vi "Pack6_UNDT.vi"(0 "data_in":u8[](array[numeric])=[86, 52, 18, 120, 86, 52, 18, 2, 0, 0, 0, 112, 204, 67, 22, 156, 119, 190, 97, 0, 16, 0, 139, 0, 0, 0, 0, 0, 0, 0, 0, 0, 0, 0, 0, 0, 0, 0, 0, 0, 0, 0, 0, 111, 18, 131, 57, 0, 0, 0, 0, 0, 1, 0, 1, 43, 25, 0, 1, 255, 255, 34, 34, 255, 255, 255, 255, 255, 255, 255, 255, 255, 255, 255, 255, 255, 255, 255, 255, 255, 255, 255, 255, 255, 255, 255, 255, 255, 255, 255, 255, 255, 255, 255, 255, 255, 255, 255, 255, 255, 255, 255, 255, 255, 255, 255, 255, 255, 255, 255, 255, 255, 255, 255, 255, 255, 255, 255, 255, 255, 255, 255, 255, 120, 86, 52, 18, 1, 0, 0, 0, 112, 204, 67, 22, 156, 119, 190, 97, 0, 16, 0, 139, 0, 0, 0, 0, 0, 0, 0, 0, 0, 0, 0, 0, 0, 0, 0, 0, 0, 0, 0, 0, 111, 18, 131, 57, 0, 0, 0, 0, 0, 1, 0, 1, 43, 25, 0, 1, 255, 255, 34, 17, 255, 255, 255, 255, 255, 255, 255, 255, 255, 255, 255, 255, 255, 255, 255, 255, 255, 255, 255, 255, 255, 255, 255, 255, 255, 255, 255, 255, 255, 255, 255, 255, 255, 255, 255, 255, 255, 255, 255, 255, 255, 255, 255, 255, 255, 255, 255, 255, 255, 255, 255, 255, 255, 255, 255, 255, 255, 255, 255] format="%02x", 1 "K_scale":dbl, 5 "N tick":u8 format="%02x", 9 "OptionPACK5":T4={"MagicWordStr"="xV4\u0012", "Header size"=56, "Проверка CRC8"=TRUE, "Проверка конца пакета"=TRUE, "GainCompens"=FALSE, "GainCorrection"=[[0.0, 1.0, 2.0, 3.0, 4.0, 5.0, 6.0, 7.0, 8.0, 9.0, 10.0, 11.0, 12.0, 13.0, 14.0, 15.0, 16.0, 17.0, 18.0, 19.0, 20.0, 21.0, 22.0, 23.0, 24.0, 25.0, 26.0, 27.0, 28.0, 29.0, 30.0, 31.0, 32.0, 33.0, 34.0, 35.0, 36.0, 37.0, 38.0, 39.0, 40.0], [0.007480379377256454, 0.05961025727668039, -0.2256445449069899, -0.08477459513390878, -0.19260677802883944, -0.022395839150075085, -0.076115384746043, -0.07452129161654766, -0.012380415371210218, 0.012737541388962995, 0.06895372697540661, 0.015013157866332921, -0.007045606467342559, -0.029720988817163698, 0.012859755243868034, 0.014783052645341199, 0.008698262907434648, -0.0007780407280235585, 0.0004171488690068028, 0.02092967406906331, 0.0018566195042745877, 0.009729465944000381, 0.007879136597780506, 0.028348095755020803, 0.01788279432686344, 0.01316889208220224, 0.008960543359635798, 0.01306464703510712, 0.03262709696783729, 0.0012714692473612531, -0.03761892820570949, -0.0316523389742032, 0.008159355326511571, 0.0081809109877908, 0.03836815904439456, 0.06681584703351648, 0.06544874790085742, 0.08623523673581365, 0.06010176834536063, 0.06195241245042141, 0.05245036073698361], [0.0, 0.0, 0.0, 0.0, 0.0, 0.0, 0.0, 0.0, 0.0, 0.0, 0.0, 0.0, 0.0, 0.0, 0.0, 0.0, 0.0, 0.0, 0.0, 0.0, 0.0, 0.0, 0.0, 0.0, 0.0, 0.0, 0.0, 0.0, 0.0, 0.0, 0.0, 0.0, 0.0, 0.0, 0.0, 0.0, 0.0, 0.0, 0.0, 0.0, 0.0]], "CorCh"=[], "Неотбрасывать BadEnd пакеты"=TRUE, "Неотбрасывать BadCRC пакеты"=TRUE} {"GainCorrection" format="%_4g"}, 11 "error in":errorcluster, 12 "Привести к 1":bool, 14 "GainCoef":bool) -> (3 "offset past match":i32=4, 4 "data_out":u8[](array[numeric]), 6 "output cluster 2":T2 {"UNDT_Cluster"."Gain Coeff" format="%#_6e"; "UNDT_Cluster"."Reserve 1" format="%02x"; "UNDT_Cluster"."Mux TX/RX" format="%02x"; "UNDT_Cluster"."ScanDelay" format="%02x"; "UNDT_Cluster"."SamplingInterval" format="%#_6e"; "UNDT_Cluster"."Lose Packet" format="%08x"; "UNDT_Cluster"."EncodersParam2" format="%016x"; "UNDT_Cluster"."EncodersParam1" format="%016x"; "UNDT_Cluster"."CRC 8" format="%02x"; "UNDT_Cluster"."N chanel" format="%02x"; "UNDT_Cluster"."N tick" format="%02x"; "UNDT_Cluster"."Ncycle" format="%04x"; "UNDT_Cluster"."FrameFormatVersion" format="%02x"; "UNDT_Cluster"."MagicWord" format="%.0x"}, 8 "Status":T1={"CRC8Good"=TRUE, "PackEndGood"=TRUE, "MWFind"=TRUE, "PackToSmall"=FALSE, "offset"=4}, 10 "PackToSmall":bool, 15 "error out":errorcluster)   [LabVIEW 2017]
uses:
  Control_EU/UNDT_ClusterPackRevers (Type).ctl
  Control_EU/DataCluster.ctl
  Control_EU/OptionPACK5.ctl
  Control_EU/Status_pack5.ctl
panel:
  out "magic_word":u8[](array[numeric])
  out "OfsetEndPack":i32
  out "MWFind":bool=TRUE
  out "Проверка конца пакета":bool=TRUE
  out "PackEndGood":bool=TRUE
  out "Проверка CRC8":bool=TRUE
  out "CRC8Good":bool=TRUE
  out "Header size":u32=56
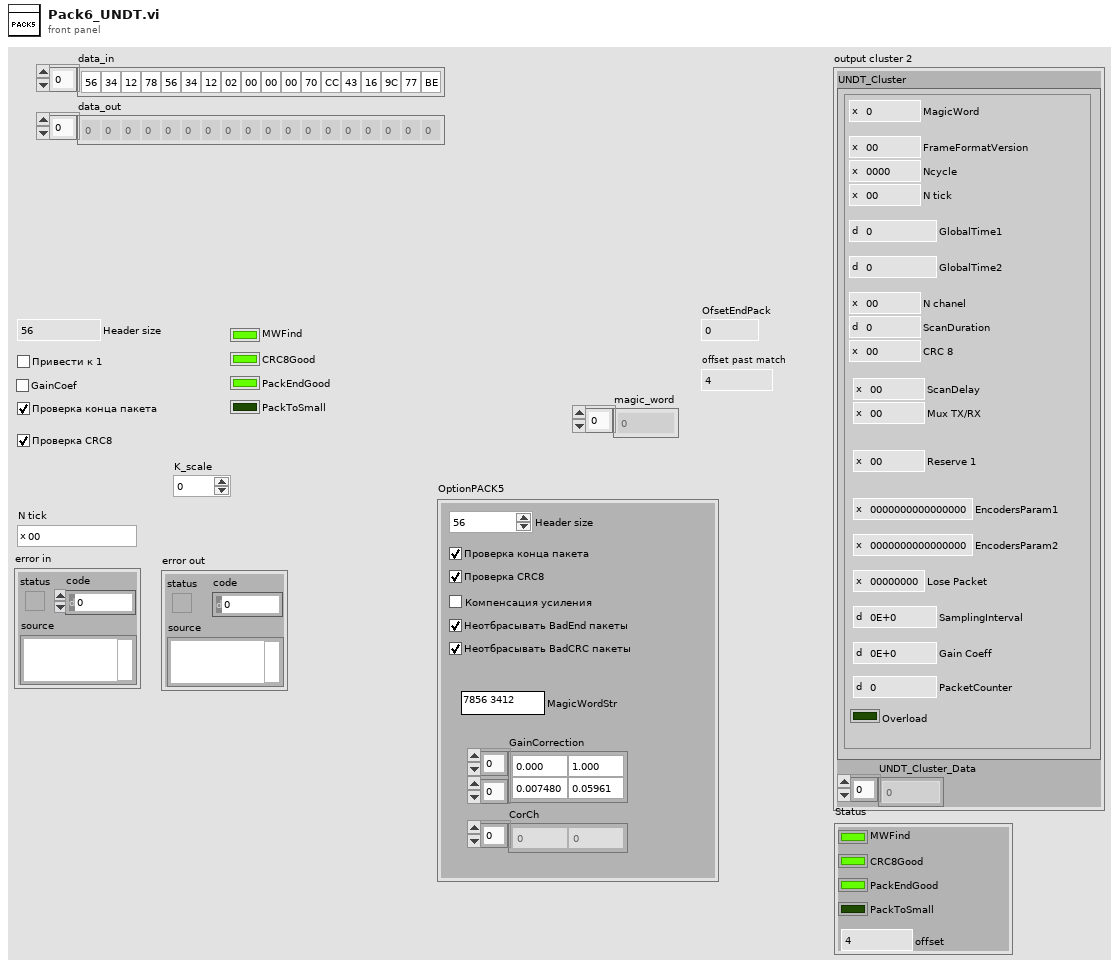
[diagram p1: front panel]
types:
  T1 = typedef "Status_pack5.ctl" = cluster{"CRC8Good":bool, "PackEndGood":bool, "MWFind":bool, "PackToSmall":bool, "offset":i32}
  T2 = typedef "DataCluster.ctl" = cluster{"UNDT_Cluster":T3, "UNDT_Cluster_Data":dbl[]}
  T3 = typedef "UNDT_ClusterPackRevers (Type).ctl" = cluster{"PacketCounter":u32, "Gain Coeff":sgl, "SamplingInterval":sgl, "Lose Packet":u32, "EncodersParam2":u64, "EncodersParam1":u64, "Reserve 1":u8, "Mux TX/RX":u8, "ScanDelay":u16, "CRC 8":u8, "ScanDuration":u16, "N chanel":u8, "GlobalTime2":u32, "GlobalTime1":u32, "N tick":u8, "Ncycle":u16, "FrameFormatVersion":u8, "MagicWord":u32, "Overload":bool}
  T4 = typedef "OptionPACK5.ctl" = cluster{"MagicWordStr":string, "Header size":u32, "Проверка CRC8":bool, "Проверка конца пакета":bool, "GainCompens":bool, "GainCorrection":dbl[][], "CorCh":dbl[], "Неотбрасывать BadEnd пакеты":bool, "Неотбрасывать BadCRC пакеты":bool}
  T5 = cluster{"CRC8Good":bool, "PackEndGood":bool, "MWFind":bool, "PackToSmall":bool, "offset past match":i32}
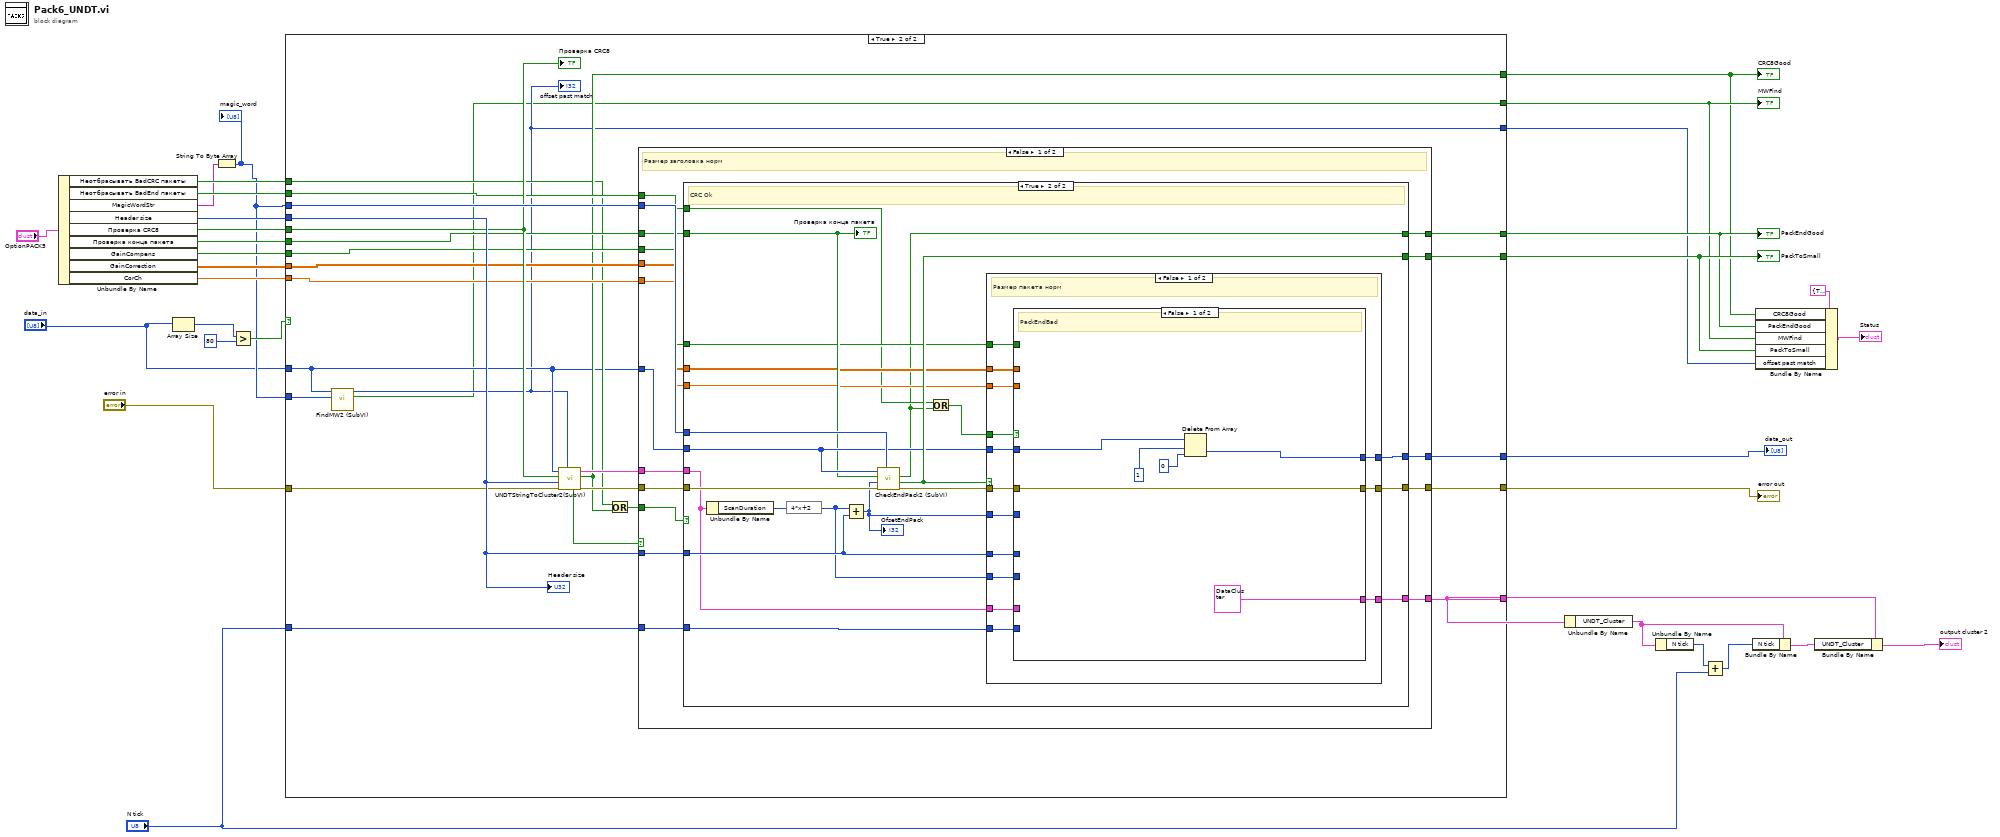
[diagram p0: block diagram]
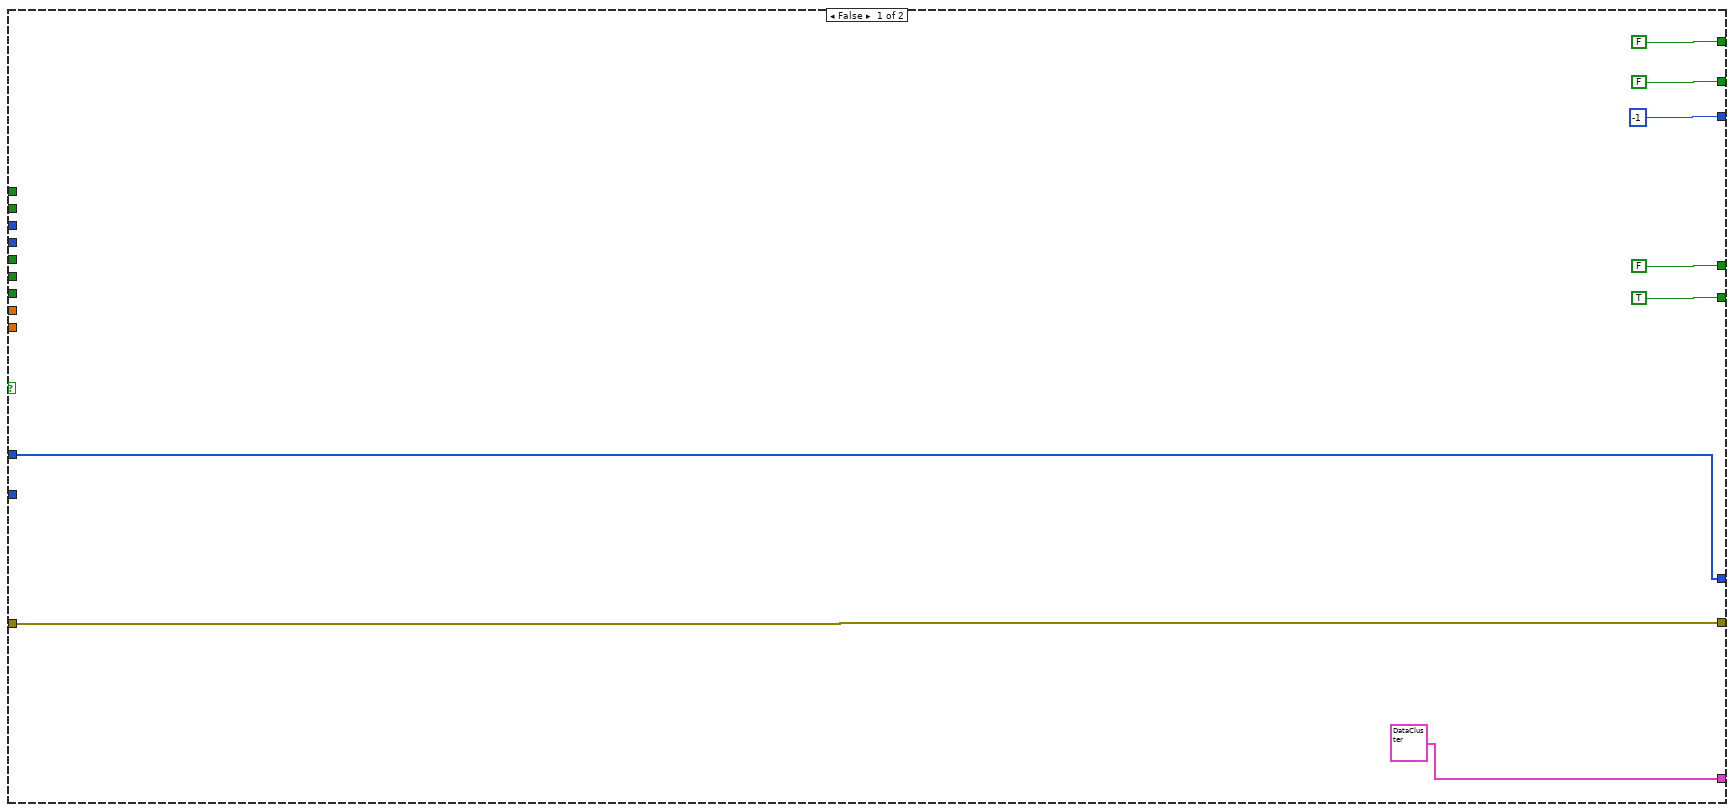
[diagram p2: hidden frame]
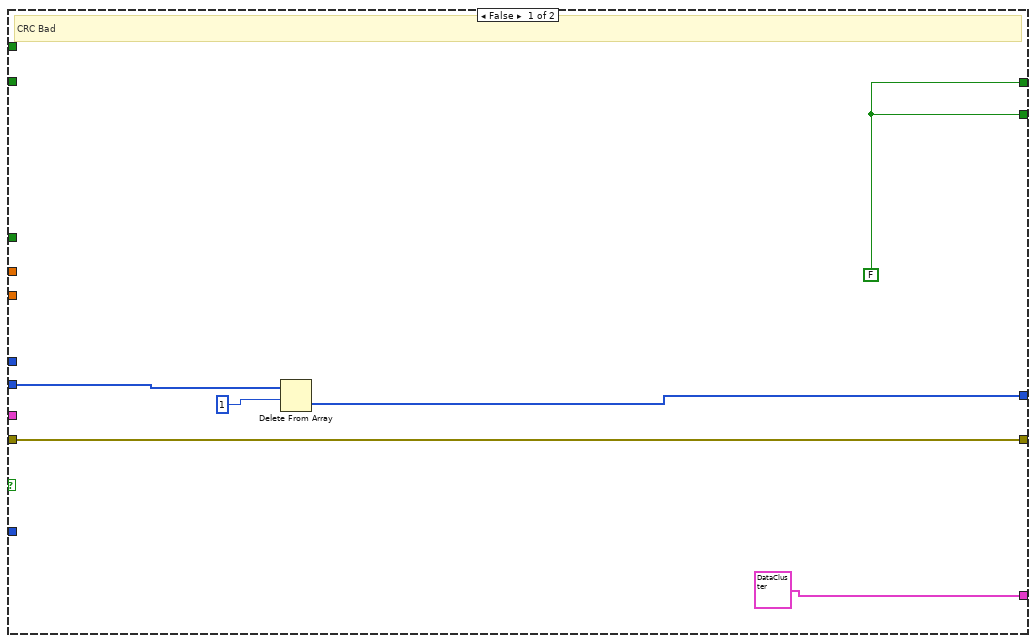
[diagram p3: hidden frame]
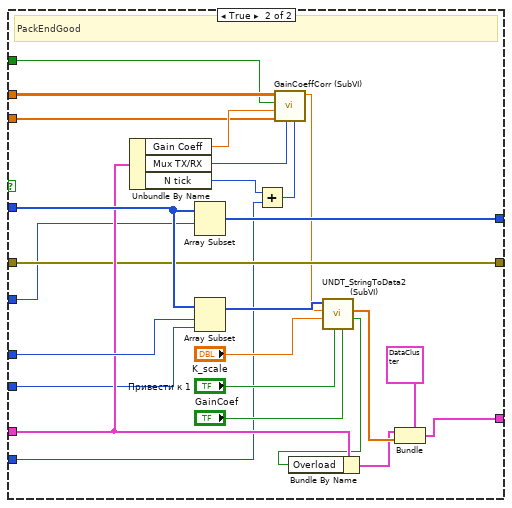
[diagram p4: hidden frame]
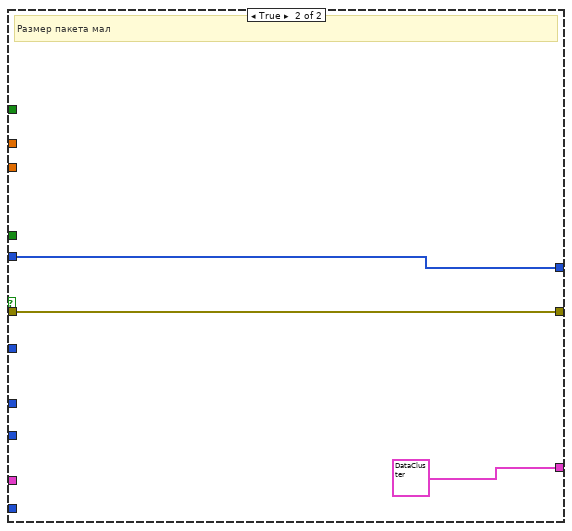
[diagram p5: hidden frame]
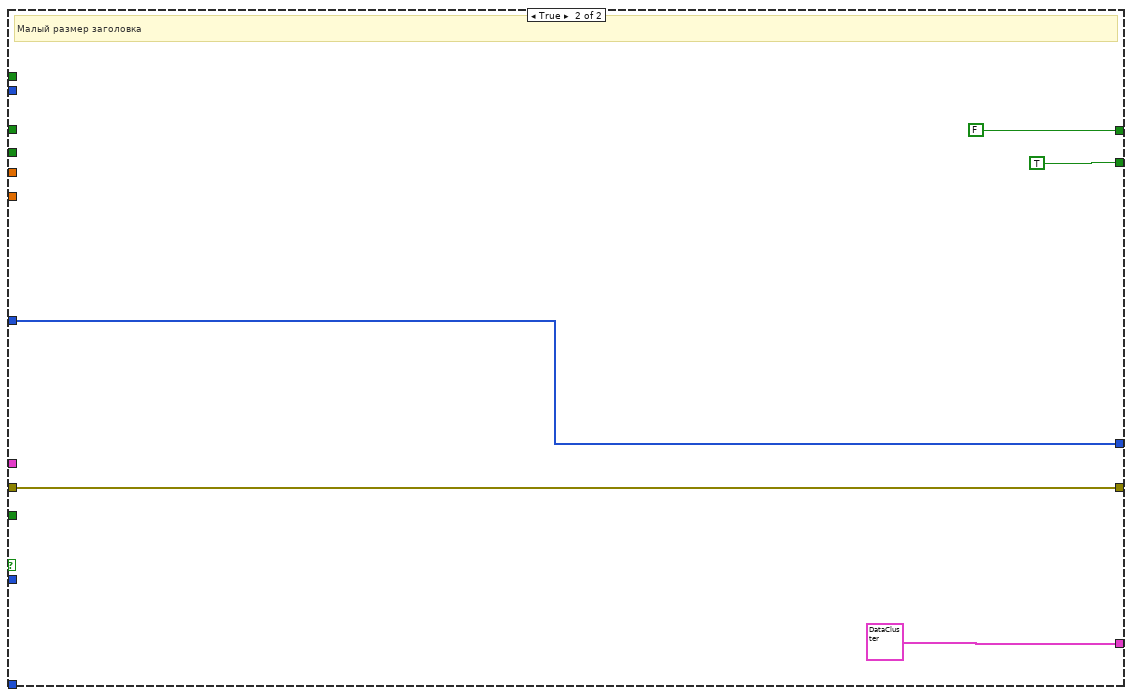
[diagram p6: hidden frame]
diagram:
  n1 = Unbundle By Name("OptionPACK5") -> ("Неотбрасывать BadCRC пакеты"=w9:bool, "Неотбрасывать BadEnd пакеты"=w11:bool, "MagicWordStr"=w4:string, "Header size"=w29:u32, "Проверка CRC8"=w28:bool, "Проверка конца пакета"=w27:bool, "GainCompens"=w20:bool, "GainCorrection"=w19:dbl[][], "CorCh"=w18:dbl[])
  n2 = Array Size(array="data_in") -> (size(s)=w5:i32)
  n3 = String To Byte Array(string=w4) -> (unsigned byte array=w2:u8[])
  "magic_word" <- w2
  n4 = Greater?(x=w5, y=80) -> (0:w6:bool)
  n5 = case shown="True" w6 {
    tunnel: [w36 w63] -> w3
    tunnel: "error in" -> [w35 w41]
    tunnel: [w35 w62] -> w31
    tunnel: w2 -> [_ w61]
    tunnel: w29 -> [_ w60]
    tunnel: w28 -> [_ w59]
    tunnel: w27 -> [_ w58]
    tunnel: [T2 {"UNDT_Cluster"={"PacketCounter"=0, "Gain Coeff"=0.0, "SamplingInterval"=0.0, "Lose Packet"=0, "EncodersParam2"=0, "EncodersParam1"=0, "Reserve 1"=0, "Mux TX/RX"=0, "ScanDelay"=0, "CRC 8"=0, "ScanDuration"=0, "N chanel"=0, "GlobalTime2"=0, "GlobalTime1"=0, "N tick"=0, "Ncycle"=0, "FrameFormatVersion"=0, "MagicWord"=0, "Overload"=FALSE}, "UNDT_Cluster_Data"=[]} ("output cluster 2") w56] -> w25
    tunnel: w20 -> [_ w55]
    tunnel: w19 -> [_ w54]
    tunnel: w18 -> [_ w53]
    tunnel: [TRUE ("PackToSmall") w52] -> w15
    tunnel: [FALSE ("PackEndGood") w51] -> w14
    tunnel: [FALSE ("MWFind") w42] -> w13
    tunnel: [-1 ("offset past match") w43] -> w12
    tunnel: w11 -> [_ w50]
    tunnel: [FALSE ("CRC8Good") w49] -> w10
    tunnel: w9 -> [_ w47]
    tunnel: "data_in" -> [w36 w44]
    tunnel: "N tick" -> [_ w46]
    tunnel: w2 -> [_ w45]
    frame False {
    }
    frame True {
      n6 = call "FindMW2 (SubVI).vi"("magic_word"=w45, "data_in"=w44) -> ("MWFind"=w42:bool, "Numeric"=w43:i32)  [unwired: 8 in]
      "offset past match" <- w43
      n7 = call "UNDTStringToCluster2(SubVI).vi"("index"=w43, "error in"=w41, "Header size"=w60, "Проверка CRC8"=w59, "data_in"=w44) -> ("error out"=w64:errorcluster, "CRC8Good"=w49:bool, "UNDT_Cluster 3"=w57:T3, "SizeToSmall"=w65:bool)  [unwired: 3 in]
      n8 = Or(x=w47, y=w49) -> (x .or. y?=w48:bool)
      n9 = case shown="False" w65 {
        tunnel: w60 -> [w82 _]
        tunnel: w61 -> [w81 _]
        tunnel: w64 -> [w80 w161]
        tunnel: w57 -> [w79 _]
        tunnel: w44 -> [w78 w162]
        tunnel: [w76 w162] -> w63
        tunnel: [w75 w161] -> w62
        tunnel: w48 -> [w77 _]
        tunnel: [w74 T2 {"UNDT_Cluster"={"PacketCounter"=0, "Gain Coeff"=0.0, "SamplingInterval"=0.0, "Lose Packet"=0, "EncodersParam2"=0, "EncodersParam1"=0, "Reserve 1"=0, "Mux TX/RX"=0, "ScanDelay"=0, "CRC 8"=0, "ScanDuration"=0, "N chanel"=0, "GlobalTime2"=0, "GlobalTime1"=0, "N tick"=0, "Ncycle"=0, "FrameFormatVersion"=0, "MagicWord"=0, "Overload"=FALSE}, "UNDT_Cluster_Data"=[]} ("output cluster 2")] -> w56
        tunnel: [w73 FALSE ("PackEndGood")] -> w51
        tunnel: [w72 TRUE ("PackToSmall")] -> w52
        tunnel: w58 -> [w71 _]
        tunnel: w55 -> [w70 _]
        tunnel: w54 -> [w69 _]
        tunnel: w46 -> [w68 _]
        tunnel: w53 -> [w67 _]
        tunnel: w50 -> [w66 _]
        frame False {
          # "Размер заголовка норм"
          n10 = case shown="True" w77 {
            tunnel: w82 -> [_ w109]
            tunnel: w81 -> [_ w100]
            tunnel: w80 -> [w85 w107]
            tunnel: w79 -> [_ w106]
            tunnel: w78 -> [w88 w99]
            tunnel: [w86 w104] -> w76
            tunnel: [w85 w103] -> w75
            tunnel: [T2 {"UNDT_Cluster"={"PacketCounter"=0, "Gain Coeff"=0.0, "SamplingInterval"=0.0, "Lose Packet"=0, "EncodersParam2"=0, "EncodersParam1"=0, "Reserve 1"=0, "Mux TX/RX"=0, "ScanDelay"=0, "CRC 8"=0, "ScanDuration"=0, "N chanel"=0, "GlobalTime2"=0, "GlobalTime1"=0, "N tick"=0, "Ncycle"=0, "FrameFormatVersion"=0, "MagicWord"=0, "Overload"=FALSE}, "UNDT_Cluster_Data"=[]} ("output cluster 2") w102] -> w74
            tunnel: [w84 w89] -> w73
            tunnel: [w84 w101] -> w72
            tunnel: w71 -> [_ w98]
            tunnel: w70 -> [_ w96]
            tunnel: w69 -> [_ w95]
            tunnel: w68 -> [_ w94]
            tunnel: w67 -> [_ w93]
            tunnel: w66 -> [_ w90]
            frame False {
              w84 = FALSE ("PackEndGood")
              # "CRC Bad"
              n11 = Delete From Array(array=w88, length=1 ("offset (0)")) -> (deleted portion=w86:u8[])  [unwired: 1 in, 1 out]
            }
            frame True {
              # "CRC Ok"
              n12 = Unbundle By Name(w106) -> ("ScanDuration"=w97:u16)
              n13 = expression code="4*x+2"(w97) -> (w108:u16)
              n14 = Add(x=w108, y=w109) -> (x+y=w92:u32)
              "OfsetEndPack" <- w92
              n15 = call "CheckEndPack2 (SubVI).vi"("magic_word"=w100, "error in"=w107, "OfsetEndPack"=w92, "Проверка конца пакета"=w98, "unsigned byte array"=w99) -> ("error out"=w105:errorcluster, "PackToSmall"=w101:bool, "PackEndGood"=w89:bool)  [unwired: 4 in]
              n16 = Or(x=w90, y=w89) -> (x .or. y?=w91:bool)
              n17 = case shown="False" w101 {
                tunnel: w109 -> [w123 _]
                tunnel: w108 -> [w122 _]
                tunnel: w106 -> [w121 _]
                tunnel: w99 -> [w120 w156]
                tunnel: w105 -> [w119 w157]
                tunnel: [w118 w156] -> w104
                tunnel: [w117 w157] -> w103
                tunnel: w91 -> [w116 _]
                tunnel: [w115 T2 {"UNDT_Cluster"={"PacketCounter"=0, "Gain Coeff"=0.0, "SamplingInterval"=0.0, "Lose Packet"=0, "EncodersParam2"=0, "EncodersParam1"=0, "Reserve 1"=0, "Mux TX/RX"=0, "ScanDelay"=0, "CRC 8"=0, "ScanDuration"=0, "N chanel"=0, "GlobalTime2"=0, "GlobalTime1"=0, "N tick"=0, "Ncycle"=0, "FrameFormatVersion"=0, "MagicWord"=0, "Overload"=FALSE}, "UNDT_Cluster_Data"=[]} ("output cluster 2")] -> w102
                tunnel: w96 -> [w114 _]
                tunnel: w95 -> [w113 _]
                tunnel: w94 -> [w112 _]
                tunnel: w93 -> [w111 _]
                tunnel: w92 -> [w110 _]
                frame False {
                  # "Размер пакета норм"
                  n18 = case shown="False" w116 {
                    tunnel: w123 -> [_ w154]
                    tunnel: w122 -> [_ w130]
                    tunnel: w121 -> [_ w146]
                    tunnel: w120 -> [w129 w153]
                    tunnel: w119 -> [w127 w141]
                    tunnel: [w128 w152] -> w118
                    tunnel: [w127 w141] -> w117
                    tunnel: [T2 {"UNDT_Cluster"={"PacketCounter"=0, "Gain Coeff"=0.0, "SamplingInterval"=0.0, "Lose Packet"=0, "EncodersParam2"=0, "EncodersParam1"=0, "Reserve 1"=0, "Mux TX/RX"=0, "ScanDelay"=0, "CRC 8"=0, "ScanDuration"=0, "N chanel"=0, "GlobalTime2"=0, "GlobalTime1"=0, "N tick"=0, "Ncycle"=0, "FrameFormatVersion"=0, "MagicWord"=0, "Overload"=FALSE}, "UNDT_Cluster_Data"=[]} ("output cluster 2") w150] -> w115
                    tunnel: w114 -> [_ w138]
                    tunnel: w113 -> [_ w140]
                    tunnel: w112 -> [_ w132]
                    tunnel: w111 -> [_ w135]
                    tunnel: w110 -> [_ w131]
                    frame False {
                      # "PackEndBad"
                      n19 = Delete From Array(array=w129, length=1 ("offset (0)"), index=0) -> (deleted portion=w128:u8[])  [unwired: 1 out]
                    }
                    frame True {
                      # "PackEndGood"
                      n20 = Unbundle By Name(w146) -> ("Gain Coeff"=w139:sgl, "Mux TX/RX"=w136:u8, "N tick"=w134:u8)
                      n21 = Array Subset(array=w153, index=w131) -> (w152:u8[])  [unwired: 1 in]
                      n22 = Array Subset(array=w153, index=w154, length=w130) -> (w148:u8[])
                      n23 = Add(x=w134, y=w132) -> (x+y=w133:u8)
                      n24 = call "GainCoeffCorr (SubVI).vi"("N tick"=w133, "ChN"=w136, "CorCh"=w135, "Gain Coeff"=w139, "GainCompens"=w138, "CorGain"=w140) -> ("Gain Coeff Corr"=w137:dbl)  [unwired: 5 in]
                      n25 = call "UNDT_StringToData2 (SubVI).vi"("GainCoef"="GainCoef", "Привести к 1"="Привести к 1", "K_scale"="K_scale", "Gain Coeff Corr"=w137, "data_in"=w148) -> ("Over"=w144:bool, "DataOut"=w151:dbl[])  [unwired: 5 in]
                      n26 = Bundle By Name(cluster=w146, "Overload"=w144) -> (w145:T3)
                      n27 = Bundle(cluster=T2 {"UNDT_Cluster"={"PacketCounter"=0, "Gain Coeff"=0.0, "SamplingInterval"=0.0, "Lose Packet"=0, "EncodersParam2"=0, "EncodersParam1"=0, "Reserve 1"=0, "Mux TX/RX"=0, "ScanDelay"=0, "CRC 8"=0, "ScanDuration"=0, "N chanel"=0, "GlobalTime2"=0, "GlobalTime1"=0, "N tick"=0, "Ncycle"=0, "FrameFormatVersion"=0, "MagicWord"=0, "Overload"=FALSE}, "UNDT_Cluster_Data"=[]} ("output cluster 2"), "UNDT_Cluster"=w145, "UNDT_Cluster_Data"=w151) -> (w150:T2)
                    }
                  }
                }
                frame True {
                  # "Размер пакета мал"
                }
              }
              "Проверка конца пакета" <- w98
            }
          }
        }
        frame True {
          # "Малый размер заголовка"
        }
      }
      "Header size" <- w60
      "Проверка CRC8" <- w59
    }
  }
  "CRC8Good" <- w10
  "error out" <- w31
  "MWFind" <- w13
  "PackEndGood" <- w14
  "PackToSmall" <- w15
  "data_out" <- w3
  n28 = Unbundle By Name(w25) -> ("UNDT_Cluster"=w24:T3)
  n29 = Unbundle By Name(w24) -> ("N tick"=w26:u8)
  n30 = Add(x=w26, y="N tick") -> (x+y=w23:u8)
  n31 = Bundle By Name(cluster=w24, "N tick"=w23) -> (w22:T3)
  n32 = Bundle By Name(cluster=T5 {"CRC8Good"=TRUE, "PackEndGood"=TRUE, "MWFind"=TRUE, "PackToSmall"=FALSE, "offset past match"=0} ("Status"), "CRC8Good"=w10, "PackEndGood"=w14, "MWFind"=w13, "PackToSmall"=w15, "offset past match"=w12) -> (→"Status":T5)
  n33 = Bundle By Name(cluster=w25, "UNDT_Cluster"=w22) -> (→"output cluster 2":T2)
